vi "!get_waveform_from_gps.vi"() -> ()   [LabVIEW 2017]
panel:
  out "speed waveform":waveform(dbl)
  out "trk.trkseg.trkpt":T1(array[cluster])
  out "position Graph":cluster{"X":dbl, "Y":dbl}[](graph)
  in  "GPX File Path":path
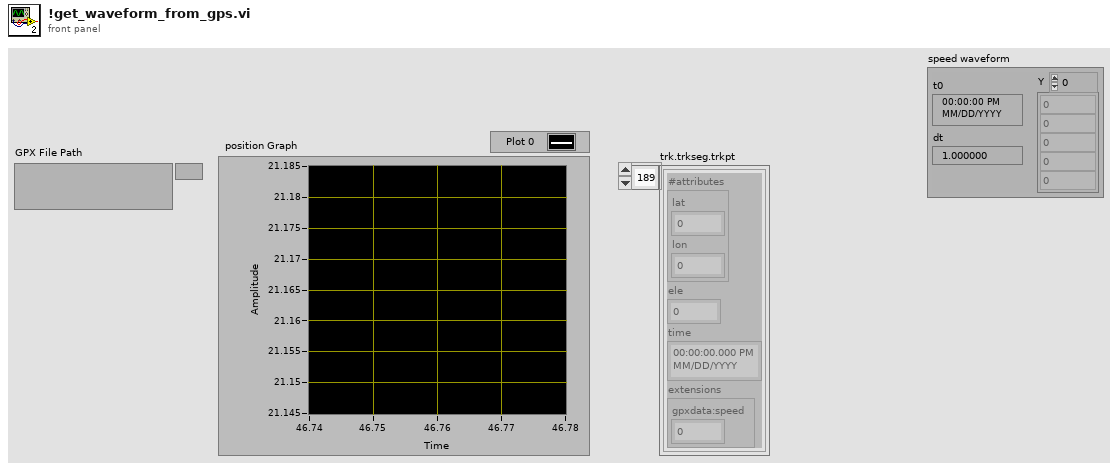
[diagram p1: front panel]
types:
  T1 = cluster{"#attributes":cluster{"lat":dbl, "lon":dbl}, "ele":dbl, "time":timestamp, "extensions":cluster{"gpxdata:speed":dbl}}[]
  T2 = cluster{"trk":cluster{"name":string, "trkseg":cluster{"trkpt":cluster{"#attributes":cluster{"lat":dbl, "lon":dbl}, "ele":dbl, "time":timestamp, "extensions":cluster{"gpxdata:speed":dbl}}[]}}}
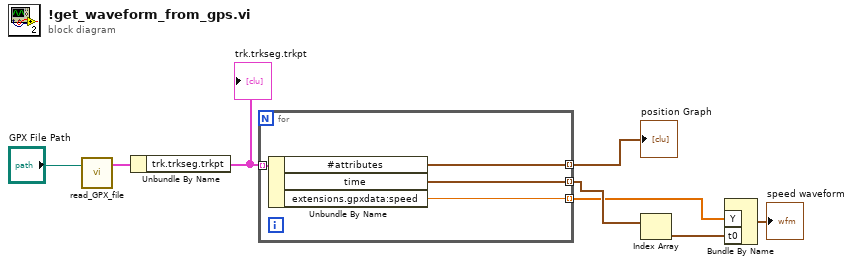
[diagram p0: block diagram]
diagram:
  n1 = call "read_GPX_file.vi"("GPX File Path"="GPX File Path") -> ("gpx data"=w6:T2)  [unwired: 1 in, 1 out]
  n2 = Unbundle By Name(w6) -> ("trk.trkseg.trkpt"=w5:T1)
  "trk.trkseg.trkpt" <- w5
  n3 = for {
    tunnel: w5 -> [w12] mode=indexing
    tunnel: [w11] -> w7 mode=indexing
    tunnel: [w10] -> w3 mode=indexing
    tunnel: [w9] -> w4 mode=indexing
    n4 = Unbundle By Name(w12) -> ("#attributes"=w11:cluster{"lat":dbl, "lon":dbl}, "time"=w9:timestamp, "extensions.gpxdata:speed"=w10:dbl)
  }
  "position Graph" <- w7
  n5 = Index Array(array=w4) -> (element=w2:timestamp)  [unwired: 1 in]
  n6 = Bundle By Name("Y"=w3, "t0"=w2) -> (→"speed waveform":waveform(dbl))  [unwired: 1 in]
